vi "Cry.vi"(8 "error in":errorcluster, 11 "Parrot in":refnum<class "Parrot.lvclass">) -> (0 "error out":errorcluster, 2 "Cry":string, 3 "Parrot out":refnum<class "Parrot.lvclass">)   [LabVIEW 2020, in "Parrot.lvclass"]
uses:
  Parrot.lvclass
  Parrot.lvclass/Parrot.ctl
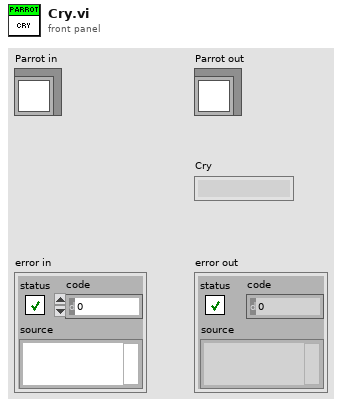
[diagram p1: front panel]
types:
  T1 = typedef "Parrot.lvclass/Parrot Type.ctl" = enum16{"European", "African", "Norwegian Blue"}
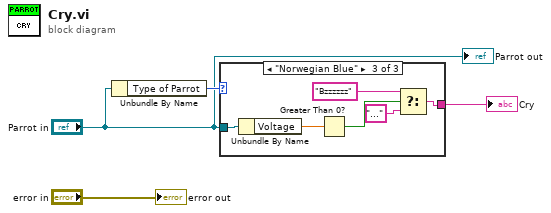
[diagram p0: block diagram]
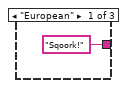
[diagram p2: hidden frame]
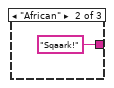
[diagram p3: hidden frame]
diagram:
  n1 = Unbundle By Name("Parrot in") -> ("Type of Parrot"=w3:T1)
  n2 = case shown="\"Norwegian Blue\"" w3 {
    tunnel: ["Sqoork!" "Sqaark!" w9] -> w2
    tunnel: "Parrot in" -> [_ _ w12]
    frame "European" {
    }
    frame "African" {
    }
    frame "Norwegian Blue" {
      n3 = Unbundle By Name(w12) -> ("Voltage"=w11:dbl)
      n4 = Greater Than 0?(x=w11) -> (x > 0?=w10:bool)
      n5 = Select(t="Bzzzzzz", s=w10, f="...") -> (s? t:f=w9:string)
    }
  }
  "Cry" <- w2
  "error out" <- "error in"
  "Parrot out" <- "Parrot in"
